vi "Polymorphic - Asynchronous Read of One JSON Message.vi"   [LabVIEW 2021]
doc: "Read a JSON message"
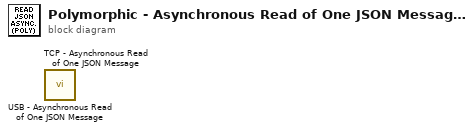
[diagram p0: block diagram]
diagram:
  n1 = call "USB - Asynchronous Read of One JSON Message.vi"() -> ()  [unwired: 9 in, 3 out]
  n2 = call "TCP - Asynchronous Read of One JSON Message.vi"() -> ()  [unwired: 9 in, 3 out]
